vi "Check If Session Valid.vi"(7 "error in (no error)":errorcluster, 10 "configuration session in":refnum<class "Configuration Session.lvclass">) -> (0 "error out":errorcluster, 2 "valid session?":bool, 3 "configuration session out":refnum<class "Configuration Session.lvclass">)   [LabVIEW 2019, in "DSF Core.lvlib" / "Configuration Session.lvclass"]
doc: "Determines whether a configuration data dsf refnum is valid."
uses:
  Configuration Session.lvclass
  Configuration Session.lvclass/Configuration Session.ctl
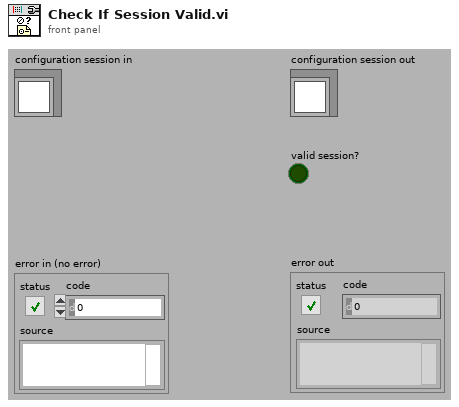
[diagram p1: front panel]
types:
  T1 = typedef "DSF Core.lvlib/Configuration Session.lvclass/DSF Config Data Ref.ctl" = refnum<data-value>
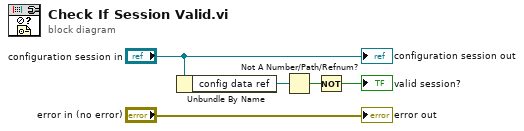
[diagram p0: block diagram]
diagram:
  n1 = Unbundle By Name("configuration session in") -> ("config data ref"=w4:T1)
  n2 = Not A Number/Path/Refnum?(number/path/refnum=w4) -> (NaN/Path/Refnum?=w5:bool)
  n3 = Not(x=w5) -> (.not. x?=→"valid session?":bool)
  "configuration session out" <- "configuration session in"
  "error out" <- "error in (no error)"
